vi "EX7-4_RC servo.vi"() -> ()   [LabVIEW 2011]
uses:
  <vilib>/LabVIEW Interface for Arduino/Type Defs/Connection Type.ctl
  <vilib>/LabVIEW Interface for Arduino/Type Defs/Board Type.ctl
  <vilib>/LabVIEW Interface for Arduino/LabVIEW Interface for Arduino.lvlib
panel:
  in  "Stop Button":bool
  out "Ready?":bool
  in  "Servo position":dbl
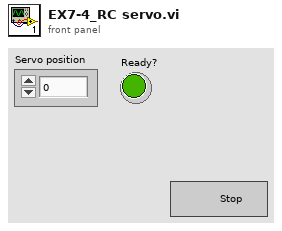
[diagram p1: front panel]
types:
  T1 = typedef "LabVIEW Interface for Arduino.lvlib/Connection Type.ctl" = enum8{"USB / Serial", "XBEE", "BlueSmirf (Bluetooth)"}
  T2 = typedef "LabVIEW Interface for Arduino.lvlib/Board Type.ctl" = enum16{"Uno", "Dimuelanove w/Atmega 328", "Mega 2560"}
  T3 = typedef "LabVIEW Interface for Arduino.lvlib/Arduino Resource.ctl" = cluster{"VISA resource":refnum<visa-resource-name>, "Board Type":T2, "Connection Type":enum8{"USB / Serial"}, "Bytes Per Packet (15)":u8}
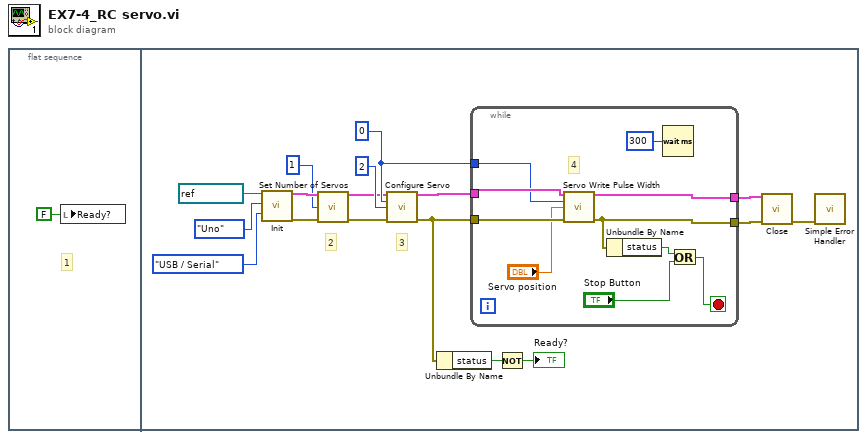
[diagram p0: block diagram]
diagram:
  n1 = flat-sequence {
    frame #0 {
      # "1"
      n2 = local write "Ready?"(FALSE ("Ready?")) -> ()
    }
    frame #1 {
      w12 = u8 0 ("Servo Number")
      # "3"
      # "2"
      n3 = call <vilib>:"Init.vi"("VISA resource"=refnum<visa-resource-name> "COM9", "Board Type (Uno)"=Board_Type."Uno", "Connection Type (USB/Serial)"=Connection_Type."USB / Serial") -> ("Arduino Resource"=w9:T3, "error out"=w6:errorcluster)  [unwired: 15 in]
      n4 = call <vilib>:"Set Number of Servos.vi"("Arduino Resource"=w9, "Number Of Servos (1)"=u8 1, "error in"=w6) -> ("Arduino Resource"=w8:T3, "error out"=w5:errorcluster)  [unwired: 11 in]
      n5 = call <vilib>:"Configure Servo.vi"("Arduino Resource"=w8, "Servo Number (0)"=w12, "DIO Pin (2)"=u8 2 ("Servo Number"), "error in"=w5) -> ("Arduino Resource"=w13:T3, "error out"=w4:errorcluster)  [unwired: 10 in]
      n6 = Unbundle By Name(w4) -> ("status"=w2:bool)
      n7 = while {
        tunnel: w13 -> [w28]
        tunnel: w4 -> [w27]
        tunnel: w12 -> [w26]
        tunnel: [w25] -> w11
        tunnel: [w22] -> w10
        stop <- w19 stop-if-true
        # "4"
        n8 = call <vilib>:"Servo Write Pulse Width.vi"("Arduino Resource"=w28, "Servo Number"=w26, "Pulse Width in uS"="Servo position", "error in"=w27) -> ("Arduino Resource"=w25:T3, "error out"=w22:errorcluster)  [unwired: 10 in]
        n9 = Unbundle By Name(w22) -> ("status"=w21:bool)
        n10 = Wait (ms)(milliseconds to wait=u32 300) -> ()  [unwired: 1 out]
        n11 = Or(x=w21, y="Stop Button") -> (x .or. y?=w19:bool)
      }
      n12 = Not(x=w2) -> (.not. x?=→"Ready?":bool)
      n13 = call <vilib>:"Close.vi"("Arduino Resource"=w11, "error in"=w10) -> ("error out"=w16:errorcluster)  [unwired: 13 in]
      n14 = call <vilib>:"Simple Error Handler.vi"("error in (no error)"=w16) -> ()  [unwired: 4 in, 5 out]
    }
  }
